vi "log_marginal_likelihood.vi"(8 "error in (no error)":errorcluster, 11 "Interface_log_marginal_likelihood in":refnum<class "Interface_log_marginal_likelihood.lvclass">) -> (0 "error out":errorcluster, 2 "out":T1, 3 "Interface_log_marginal_likelihood out":refnum<class "Interface_log_marginal_likelihood.lvclass">)   [LabVIEW 2020, in "Interface_log_marginal_likelihood.lvclass"]
doc: "Returns log-marginal likelihood of theta for training data."
uses:
  Interface_log_marginal_likelihood.lvclass
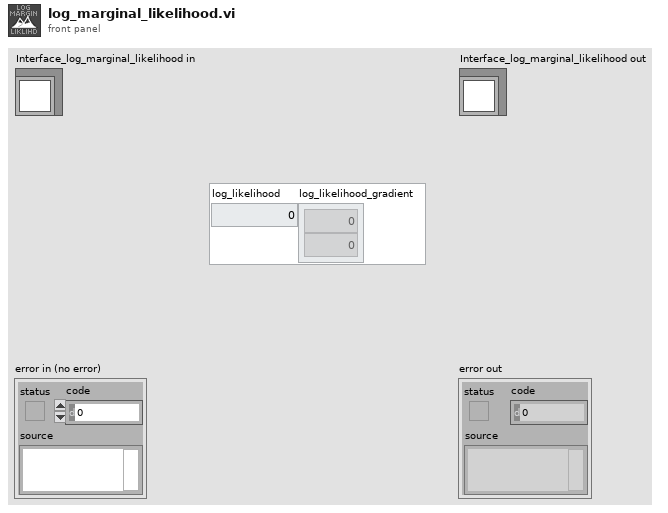
[diagram p1: front panel]
types:
  T1 = cluster{"log_likelihood":dbl, "log_likelihood_gradient":dbl[]}
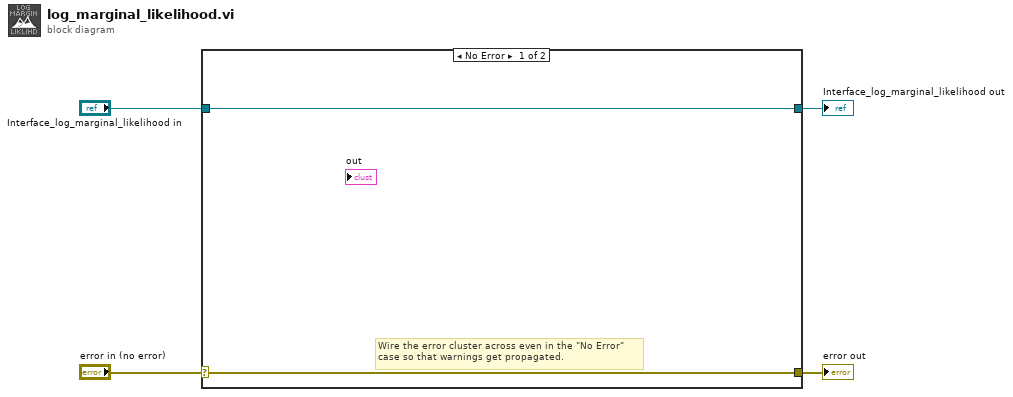
[diagram p0: block diagram]
diagram:
  n1 = case shown="No Error" "error in (no error)" {
    selector: "error in (no error)" -> [w5 w8]
    tunnel: [w5 w8] -> w3
    tunnel: [w6 w7] -> w1
    tunnel: "Interface_log_marginal_likelihood in" -> [w6 w7]
    frame No Error {
      # "Wire the error cluster across even in the \"No Error\"\ncase so that warnings get propagated."
    }
    frame Error {
    }
  }
  "error out" <- w3
  "Interface_log_marginal_likelihood out" <- w1
